vi "Test.vi"() -> ()   [LabVIEW 2015, in "Main INI.lvlib"]
uses:
  Main INI.lvlib
  Core Data.ctl
  Re-use Libraries/Utility/Utility.lvlib
panel:
  in  "Read":bool=TRUE
  out "Data out":T1
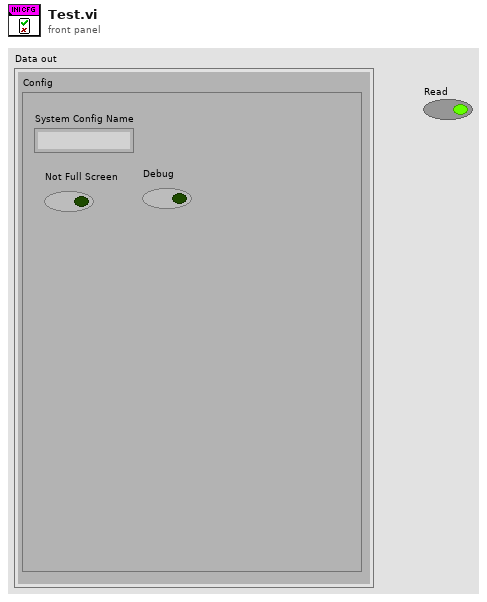
[diagram p1: front panel]
types:
  T1 = typedef "Main INI.lvlib/Core Data.ctl" = cluster{"Config":cluster{"System Config Name":string, "Not Full Screen":bool, "Debug":bool}}
  T2 = typedef "Utility.lvlib/App Paths.ctl" = cluster{"App Ini File":path, "App Data Dir":path, "Config Dir":path, "App Root Dir":path}
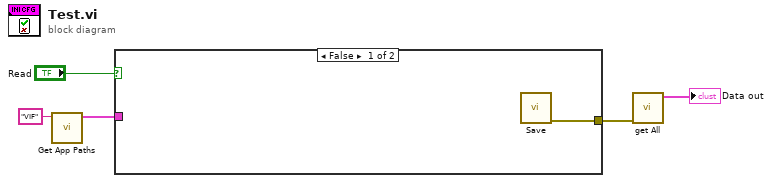
[diagram p0: block diagram]
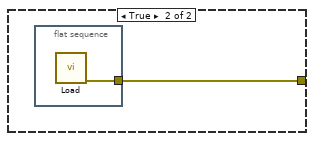
[diagram p2: hidden frame]
diagram:
  n1 = call "Get App Paths.vi"("Build Name"="VIF") -> ("Paths"=w1:T2)  [unwired: 9 in, 1 out]
  n2 = case shown="False" "Read" {
    tunnel: [w6 w7] -> w4
    tunnel: w1 -> [_ _]
    frame False {
      n3 = call "Save.vi"() -> ("error out"=w6:errorcluster)  [unwired: 11 in]
    }
    frame True {
      n4 = flat-sequence {
        tunnel: [w8] -> w7
        frame #0 {
          n5 = call "Load.vi"() -> ("error out"=w8:errorcluster)  [unwired: 10 in, 1 out]
        }
      }
    }
  }
  n6 = call "get All.vi"("error in"=w4) -> ("Data out"=→"Data out":T1)  [unwired: 9 in, 1 out]
